vi "Reset Commanding.vi"(8 "error in (no error)":errorcluster, 9 "Cmd State":T1, 11 "DblPopupControl in":refnum<class "DblPopupControl.lvclass">) -> (0 "error out":errorcluster, 3 "DblPopupControl out":refnum<class "DblPopupControl.lvclass">)   [LabVIEW 2020, in "VolatusGUIElements.lvlib" / "DblPopupControl.lvclass"]
uses:
  DblPopupControl.lvclass
  Cmd State.ctl
  DblPopupControl.lvclass/DblPopupControl.ctl
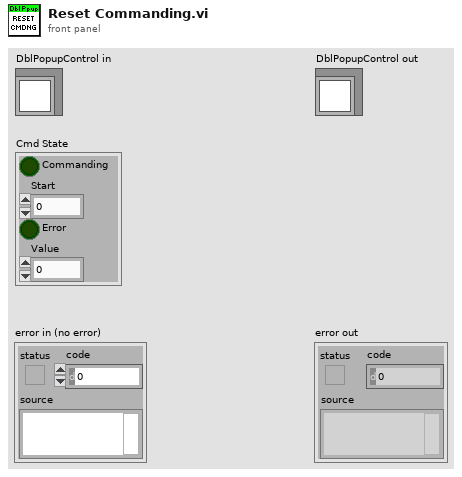
[diagram p1: front panel]
types:
  T1 = typedef "VolatusGUIElements.lvlib/DblPopupControl.lvclass/Cmd State.ctl" = cluster{"Commanding":bool, "Start":dbl, "Error":bool, "Value":dbl}
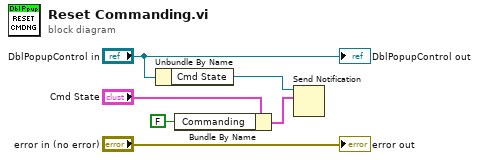
[diagram p0: block diagram]
diagram:
  n1 = Unbundle By Name("DblPopupControl in") -> ("Cmd State"=w4:refnum<notifier>)
  n2 = Bundle By Name(cluster="Cmd State", "Commanding"=FALSE) -> (w2:T1)
  n3 = Send Notification(notification=w2, notifier=w4) -> ()  [unwired: 1 in, 2 out]
  "error out" <- "error in (no error)"
  "DblPopupControl out" <- "DblPopupControl in"
